vi "HEWH PRAT Valves.vi"(8 "error in (no error)":errorcluster, 9 "Normally Open Valve":T1, 10 "Station ID":T2=enum."A", 11 "MW100 In":refnum<visa-resource-name>) -> (0 "error out":errorcluster, 3 "MW100 Out":refnum<visa-resource-name>)   [LabVIEW 2016]
uses:
  Type Definitions/Station ID Selector.ctl
  Type Definitions/HEWH Normally Open Valve Control.ctl
  Type Definitions/PRAT Channel Settings.ctl
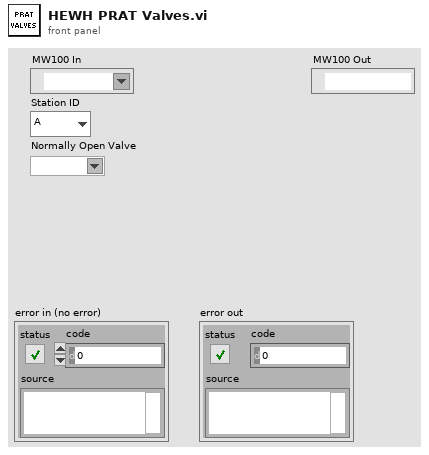
[diagram p1: front panel]
types:
  T1 = typedef "HEWH Normally Open Valve Control.ctl" = string
  T2 = typedef "Station ID Selector.ctl" = enum16{"", "A", "B", "C", "D", "Global"}
  T3 = typedef "PRAT Channel Settings.ctl" = string
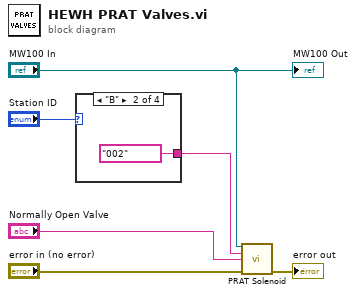
[diagram p0: block diagram]
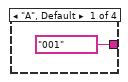
[diagram p2: hidden frame]
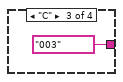
[diagram p3: hidden frame]
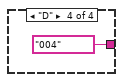
[diagram p4: hidden frame]
diagram:
  n1 = case shown="\"B\"" "Station ID" {
    tunnel: [T3 "001" ("PRAT Channels") T3 "002" ("PRAT Channels") T3 "003" ("PRAT Channels") T3 "004" ("PRAT Channels")] -> w6
    frame "A", Default {
    }
    frame "B" {
    }
    frame "C" {
    }
    frame "D" {
    }
  }
  n2 = call "PRAT Solenoid.vi"("VISA session"="MW100 In", "PRAT Channels"=w6, "Normally Open Valve"="Normally Open Valve", "Error In"="error in (no error)") -> ("Error Out"=→"error out":errorcluster)  [unwired: 10 in, 1 out]
  "MW100 Out" <- "MW100 In"
